vi "cam1analyse.vi"() -> (0 "W3 chiffre":string, 1 "W2 chiffre":string, 2 "R6 chiffre":string, 3 "W1 chiffre":string, 5 "W4 chiffre":string, 6 "B1 chiffre":string, 7 "B2 chiffre":string, 8 "R3 chiffre":string, 9 "R8 chiffre":string, 10 "B3 chiffre":string, 11 "B4 chiffre":string, 12 "B6 chiffre":string, 13 "B7 chiffre":string, 14 "B8 chiffre":string, 15 "B9 chiffre":string, 16 "R9 chiffre":string)   [LabVIEW 2019]
uses:
  <vilib>/vision/Classification.llb/IMAQ Classifier Read Options.ctl
  <vilib>/vision/NI_Vision_Development_Module.lvlib
panel:
  out "Coordinates":i32[](array[numeric])
  in  "R9":T1={"Global Rectangle"=[0, 0, 1279, 959], "Contours"=[{"ID"=enum."External", "Type"=3, "Coordinates"=[0, 0, 1279, 959]}]} {"Contours"."Type" items=["No Selection", "Point", "Line", "Rectangle", "Oval", "Polygon", "Freehand Region", "Annulus", "Unused2", "Unused3", "Broken Line", "Freehand Line", "Rotated Rectangle"]}
  out "R9 2":string[](array[string])
  in  "R8":T1={"Global Rectangle"=[0, 0, 1279, 959], "Contours"=[{"ID"=enum."External", "Type"=3, "Coordinates"=[0, 0, 1279, 959]}]} {"Contours"."Type" items=["No Selection", "Point", "Line", "Rectangle", "Oval", "Polygon", "Freehand Region", "Annulus", "Unused2", "Unused3", "Broken Line", "Freehand Line", "Rotated Rectangle"]}
  out "R8 2":string[](array[string])
  in  "R6":T1={"Global Rectangle"=[0, 0, 1279, 959], "Contours"=[{"ID"=enum."External", "Type"=3, "Coordinates"=[0, 0, 1279, 959]}]} {"Contours"."Type" items=["No Selection", "Point", "Line", "Rectangle", "Oval", "Polygon", "Freehand Region", "Annulus", "Unused2", "Unused3", "Broken Line", "Freehand Line", "Rotated Rectangle"]}
  out "R6 2":string[](array[string])
  in  "R3":T1={"Global Rectangle"=[0, 0, 1279, 959], "Contours"=[{"ID"=enum."External", "Type"=3, "Coordinates"=[0, 0, 1279, 959]}]} {"Contours"."Type" items=["No Selection", "Point", "Line", "Rectangle", "Oval", "Polygon", "Freehand Region", "Annulus", "Unused2", "Unused3", "Broken Line", "Freehand Line", "Rotated Rectangle"]}
  out "R3 2":string[](array[string])
  in  "B9":T1={"Global Rectangle"=[0, 0, 1279, 959], "Contours"=[{"ID"=enum."External", "Type"=3, "Coordinates"=[0, 0, 1279, 959]}]} {"Contours"."Type" items=["No Selection", "Point", "Line", "Rectangle", "Oval", "Polygon", "Freehand Region", "Annulus", "Unused2", "Unused3", "Broken Line", "Freehand Line", "Rotated Rectangle"]}
  out "B9 2":string[](array[string])
  in  "B8":T1={"Global Rectangle"=[0, 0, 1279, 959], "Contours"=[{"ID"=enum."External", "Type"=3, "Coordinates"=[0, 0, 1279, 959]}]} {"Contours"."Type" items=["No Selection", "Point", "Line", "Rectangle", "Oval", "Polygon", "Freehand Region", "Annulus", "Unused2", "Unused3", "Broken Line", "Freehand Line", "Rotated Rectangle"]}
  out "B8 2":string[](array[string])
  in  "B7":T1={"Global Rectangle"=[0, 0, 1279, 959], "Contours"=[{"ID"=enum."External", "Type"=3, "Coordinates"=[0, 0, 1279, 959]}]} {"Contours"."Type" items=["No Selection", "Point", "Line", "Rectangle", "Oval", "Polygon", "Freehand Region", "Annulus", "Unused2", "Unused3", "Broken Line", "Freehand Line", "Rotated Rectangle"]}
  out "B7 2":string[](array[string])
  in  "B6":T1={"Global Rectangle"=[0, 0, 1279, 959], "Contours"=[{"ID"=enum."External", "Type"=3, "Coordinates"=[0, 0, 1279, 959]}]} {"Contours"."Type" items=["No Selection", "Point", "Line", "Rectangle", "Oval", "Polygon", "Freehand Region", "Annulus", "Unused2", "Unused3", "Broken Line", "Freehand Line", "Rotated Rectangle"]}
  out "B6 2":string[](array[string])
  in  "B4":T1={"Global Rectangle"=[0, 0, 1279, 959], "Contours"=[{"ID"=enum."External", "Type"=3, "Coordinates"=[0, 0, 1279, 959]}]} {"Contours"."Type" items=["No Selection", "Point", "Line", "Rectangle", "Oval", "Polygon", "Freehand Region", "Annulus", "Unused2", "Unused3", "Broken Line", "Freehand Line", "Rotated Rectangle"]}
  out "B4 2":string[](array[string])
  in  "B3":T1={"Global Rectangle"=[0, 0, 1279, 959], "Contours"=[{"ID"=enum."External", "Type"=3, "Coordinates"=[0, 0, 1279, 959]}]} {"Contours"."Type" items=["No Selection", "Point", "Line", "Rectangle", "Oval", "Polygon", "Freehand Region", "Annulus", "Unused2", "Unused3", "Broken Line", "Freehand Line", "Rotated Rectangle"]}
  out "B3 2":string[](array[string])
  in  "B2":T1={"Global Rectangle"=[0, 0, 1279, 959], "Contours"=[{"ID"=enum."External", "Type"=3, "Coordinates"=[0, 0, 1279, 959]}]} {"Contours"."Type" items=["No Selection", "Point", "Line", "Rectangle", "Oval", "Polygon", "Freehand Region", "Annulus", "Unused2", "Unused3", "Broken Line", "Freehand Line", "Rotated Rectangle"]}
  out "B2 2":string[](array[string])
  in  "B1":T1={"Global Rectangle"=[0, 0, 1279, 959], "Contours"=[{"ID"=enum."External", "Type"=3, "Coordinates"=[0, 0, 1279, 959]}]} {"Contours"."Type" items=["No Selection", "Point", "Line", "Rectangle", "Oval", "Polygon", "Freehand Region", "Annulus", "Unused2", "Unused3", "Broken Line", "Freehand Line", "Rotated Rectangle"]}
  out "B1 2":string[](array[string])
  in  "W4":T1={"Global Rectangle"=[0, 0, 1279, 959], "Contours"=[{"ID"=enum."External", "Type"=3, "Coordinates"=[0, 0, 1279, 959]}]} {"Contours"."Type" items=["No Selection", "Point", "Line", "Rectangle", "Oval", "Polygon", "Freehand Region", "Annulus", "Unused2", "Unused3", "Broken Line", "Freehand Line", "Rotated Rectangle"]}
  out "W4 2":string[](array[string])
  in  "W1":T1={"Global Rectangle"=[0, 0, 1279, 959], "Contours"=[{"ID"=enum."External", "Type"=3, "Coordinates"=[0, 0, 1279, 959]}]} {"Contours"."Type" items=["No Selection", "Point", "Line", "Rectangle", "Oval", "Polygon", "Freehand Region", "Annulus", "Unused2", "Unused3", "Broken Line", "Freehand Line", "Rotated Rectangle"]}
  out "W1 2":string[](array[string])
  in  "W2 2":T1={"Global Rectangle"=[0, 0, 1279, 959], "Contours"=[{"ID"=enum."External", "Type"=3, "Coordinates"=[0, 0, 1279, 959]}]} {"Contours"."Type" items=["No Selection", "Point", "Line", "Rectangle", "Oval", "Polygon", "Freehand Region", "Annulus", "Unused2", "Unused3", "Broken Line", "Freehand Line", "Rotated Rectangle"]}
  out "W2 3":string[](array[string])
  in  "W3":T1={"Global Rectangle"=[640, 450, 686, 504], "Contours"=[{"ID"=enum."External", "Type"=3, "Coordinates"=[640, 450, 686, 504]}]} {"Contours"."Type" items=["No Selection", "Point", "Line", "Rectangle", "Oval", "Polygon", "Freehand Region", "Annulus", "Unused2", "Unused3", "Broken Line", "Freehand Line", "Rotated Rectangle"]}
  out "Image Out":T2(plugin-control)
  out "error out":errorcluster
  out "W3":string[](array[string])
  in  "error in":errorcluster
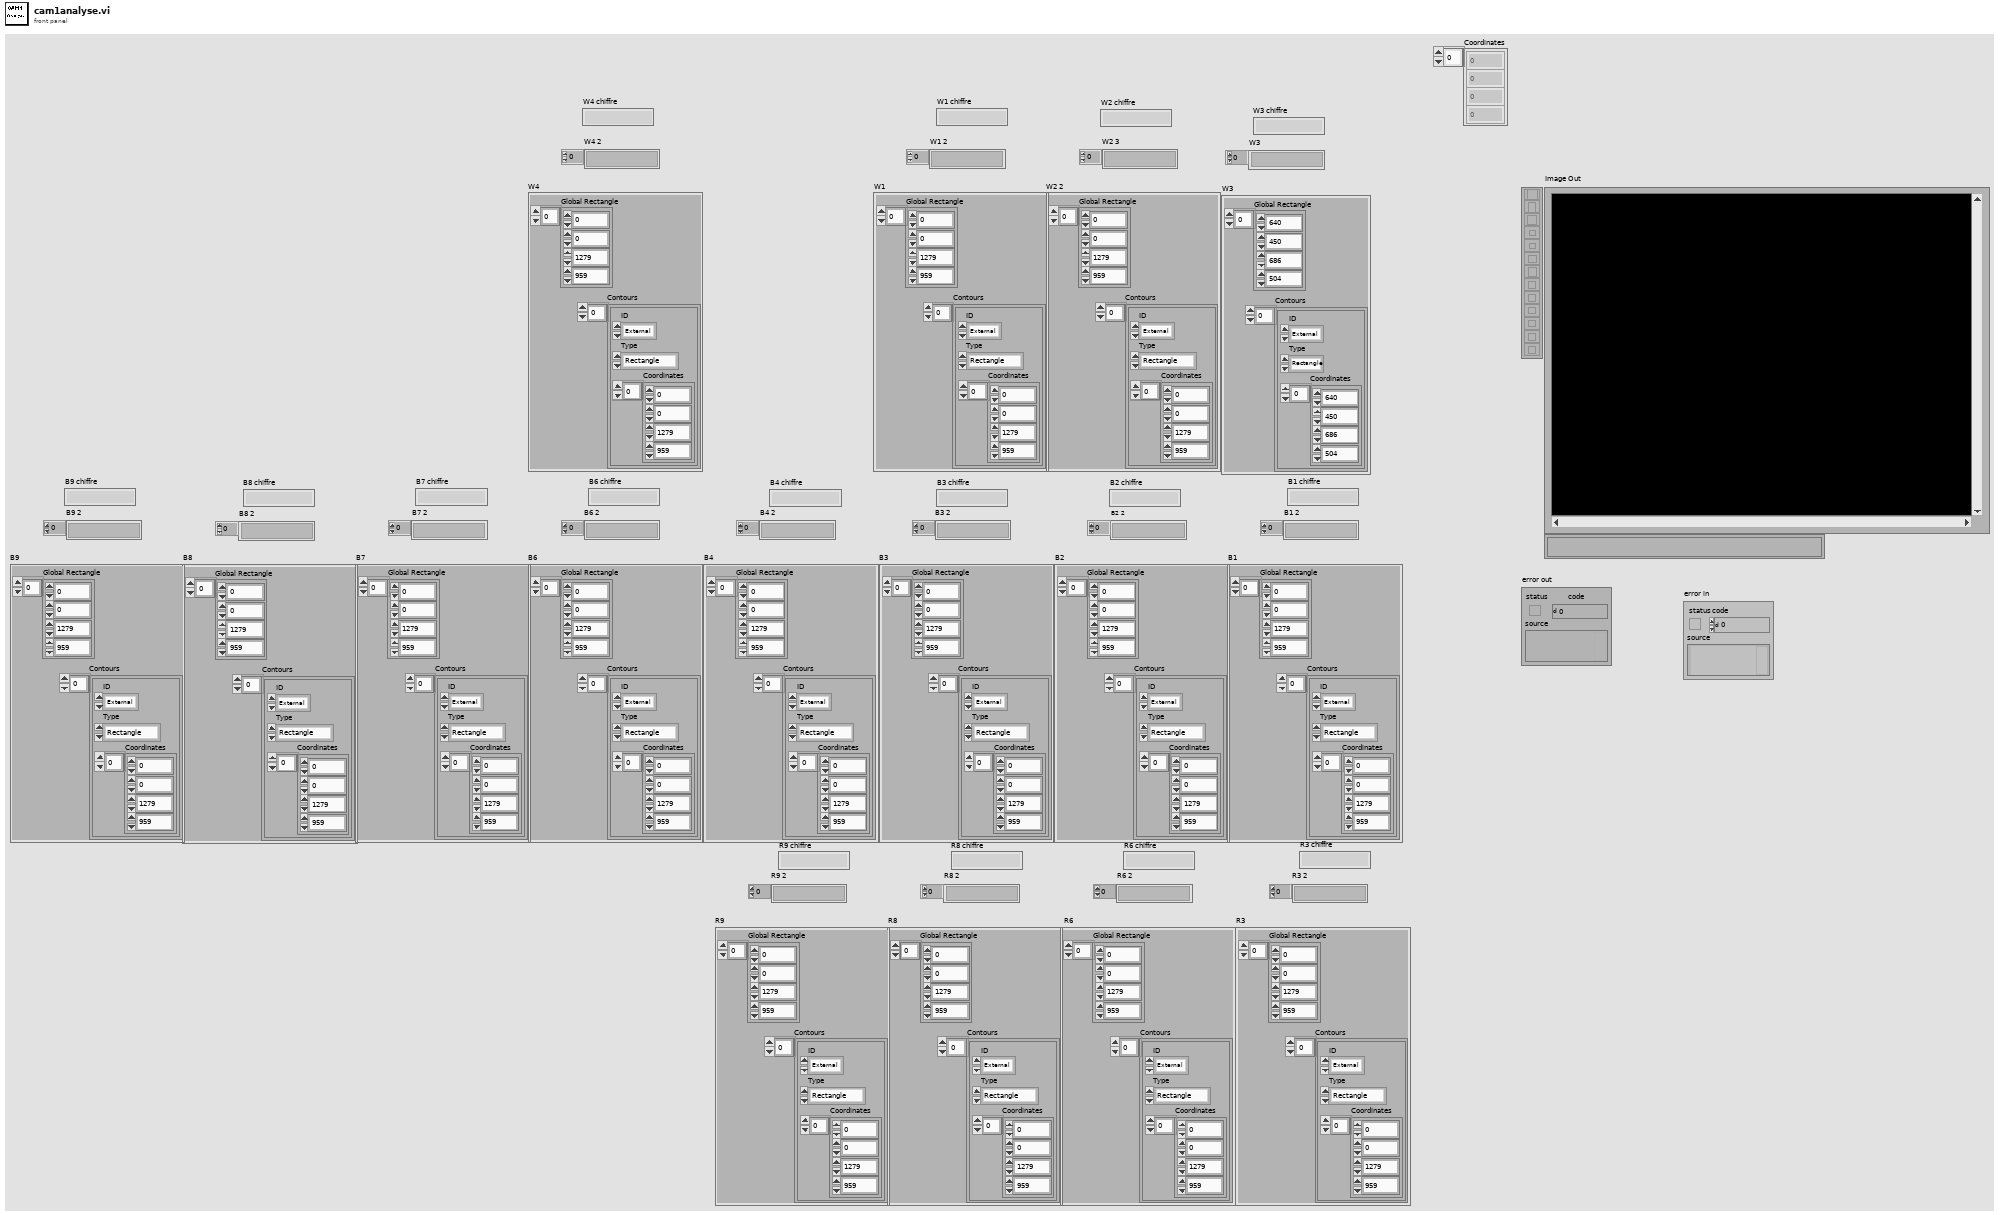
[diagram p1: front panel]
types:
  T1 = cluster{"Global Rectangle":i32[], "Contours":cluster{"ID":enum32{"External", "Internal"}, "Type":u32, "Coordinates":i32[]}[]}
  T2 = typedef "IMAQ Image.ctl" = refnum<image>
  T3 = typedef "IMAQ Classifier Read Options.ctl" = i32
  T4 = typedef "IMAQ Classifier Session.ctl" = refnum<k1>
  T5 = typedef "ROI Descriptor" = cluster{"Global Rectangle":i32[], "Contours":cluster{"ID":enum32{"External", "Internal"}, "Type":u32, "Coordinates":i32[]}[]}
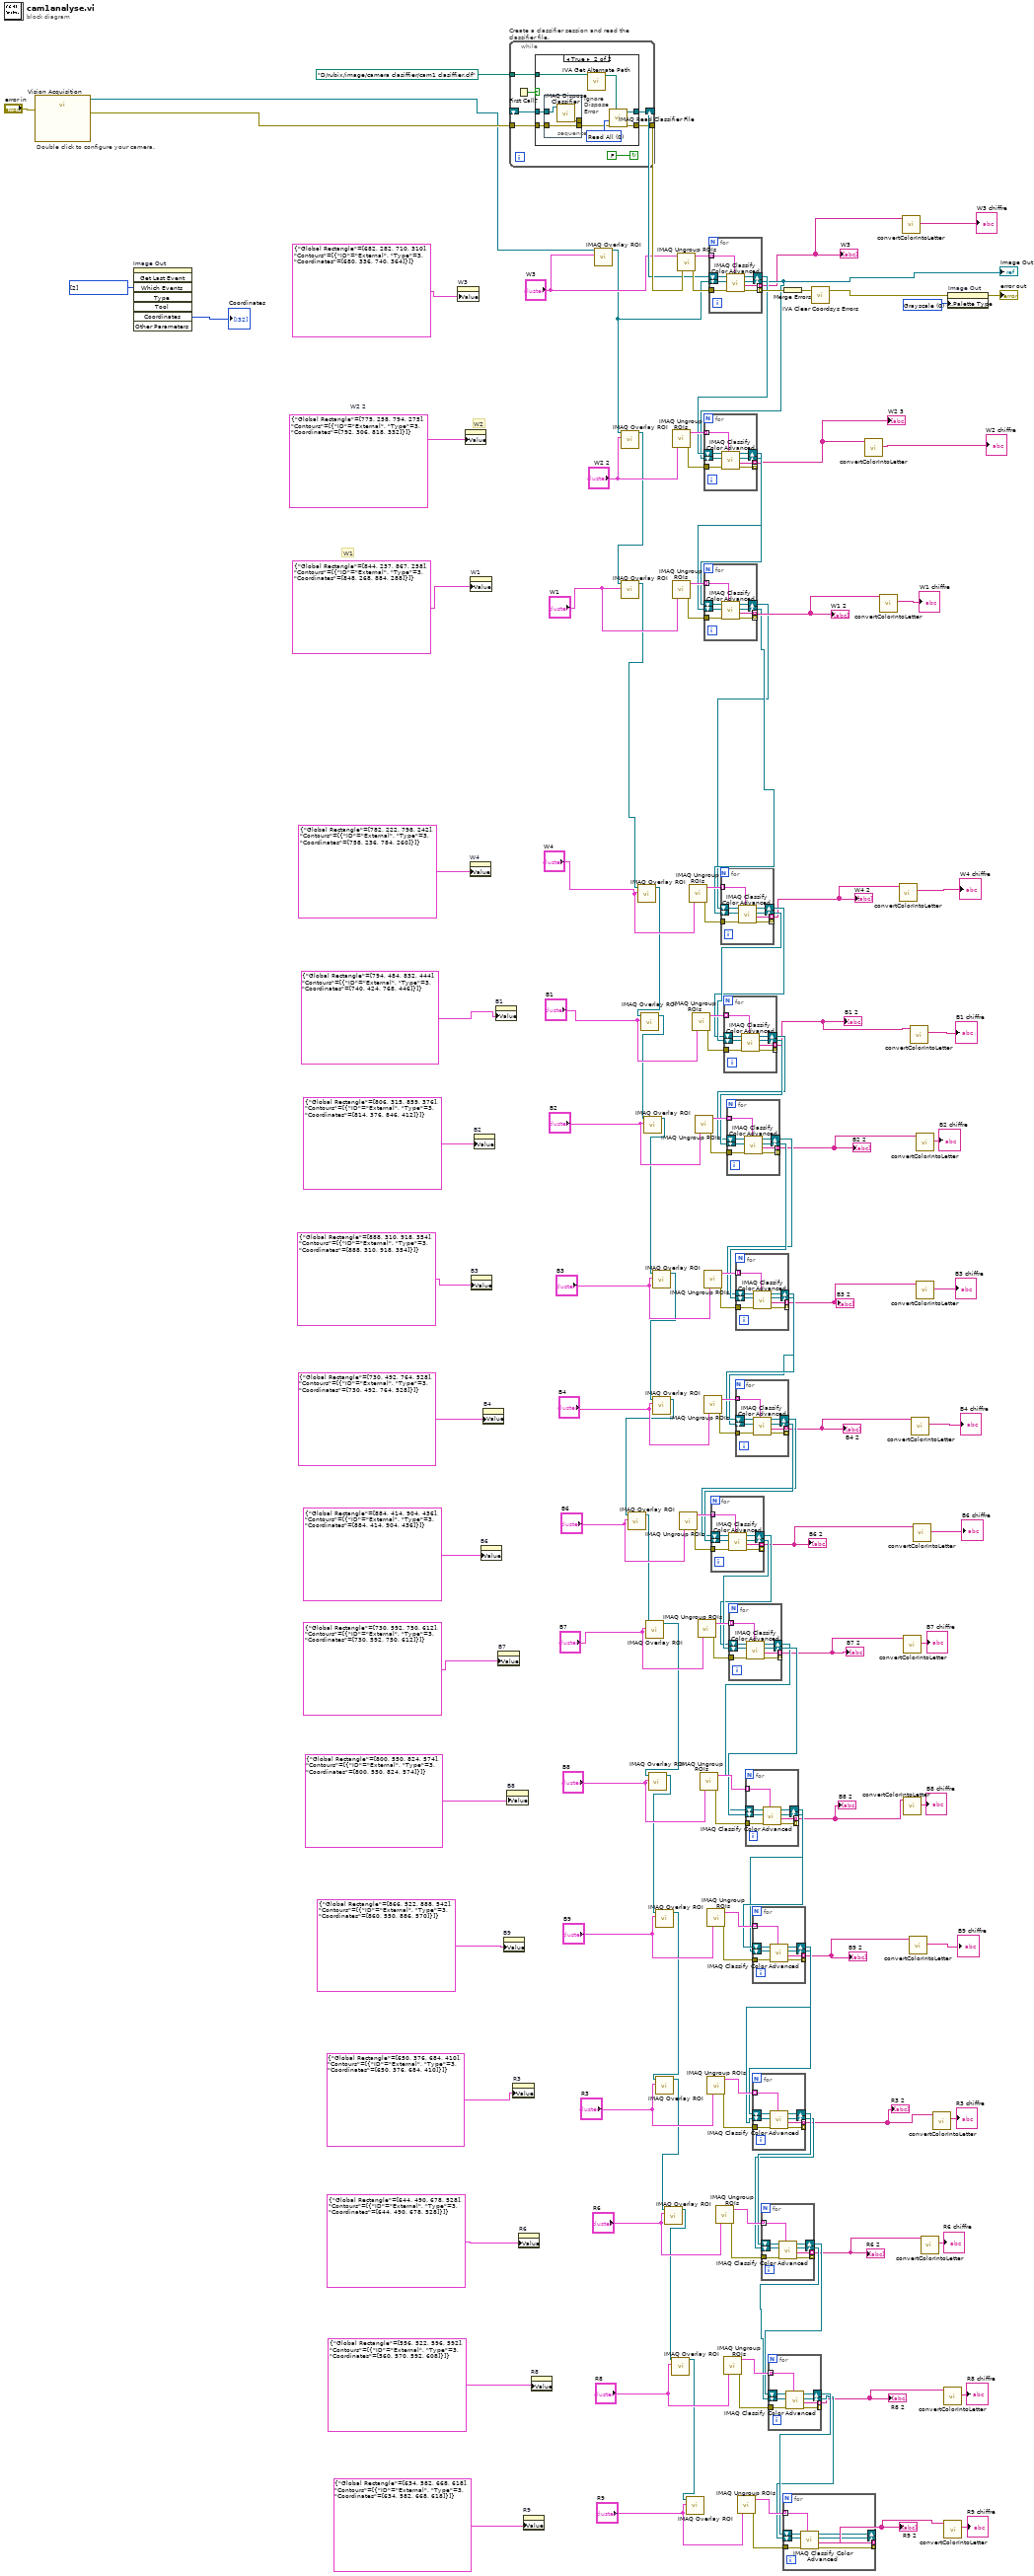
[diagram p0: block diagram]
diagram:
  w5 = i32[] [2] items=["No Event"=0, "Click Event"=1, "Draw Event"=2, "Size Event"=4, "Scroll Event"=5, "Double Click Event"=8] ("Which Events")
  w143 = u32 0 items=["Grayscale", "Binary", "Gradient", "Rainbow", "Temperature", "User Defined", "Binary 16 Bit", "Gradient 16 Bit", "Rainbow 16 Bit", "Temperature 16 Bit", "User Defined 16 Bit"] ("Palette Type")
  # "W2"
  # "W1"
  # "Double click to configure your camera."
  n1 = call "Vision Acquisition"("error in"="error in") -> ("Image Out"=w9:T2, "error out"=w153:errorcluster)  [unwired: 25 in]
  n2 = invoke on="Image Out" class="ImageControl" method="Get Last Event"("Which Events"=w5) -> ("Coordinates"=→"Coordinates":i32[])  [unwired: 7 in, 7 out]
  n3 = property on="W3" class="Clust (strict)"("Value"=T1 {"Global Rectangle"=[682, 282, 710, 310], "Contours"=[{"ID"=enum."External", "Type"=3, "Coordinates"=[680, 336, 740, 364]}]} ("ROI Descriptor (Color Classification 1)")) -> ()  [unwired: 2 in, 2 out]
  n4 = property on="W2 2" class="Clust (strict)"("Value"=T1 {"Global Rectangle"=[775, 258, 794, 275], "Contours"=[{"ID"=enum."External", "Type"=3, "Coordinates"=[792, 306, 818, 332]}]} ("ROI Descriptor (Color Classification 1)")) -> ()  [unwired: 2 in, 2 out]
  n5 = property on="W4" class="Clust (strict)"("Value"=T1 {"Global Rectangle"=[782, 222, 798, 242], "Contours"=[{"ID"=enum."External", "Type"=3, "Coordinates"=[758, 236, 784, 260]}]} ("ROI Descriptor (Color Classification 1)")) -> ()  [unwired: 2 in, 2 out]
  n6 = property on="W1" class="Clust (strict)"("Value"=T1 {"Global Rectangle"=[844, 237, 867, 258], "Contours"=[{"ID"=enum."External", "Type"=3, "Coordinates"=[848, 268, 884, 288]}]} ("ROI Descriptor (Color Classification 1)")) -> ()  [unwired: 2 in, 2 out]
  n7 = property on="B3" class="Clust (strict)"("Value"=T1 {"Global Rectangle"=[888, 310, 918, 354], "Contours"=[{"ID"=enum."External", "Type"=3, "Coordinates"=[888, 310, 918, 354]}]} ("ROI Descriptor (Color Classification 1)")) -> ()  [unwired: 2 in, 2 out]
  n8 = property on="B2" class="Clust (strict)"("Value"=T1 {"Global Rectangle"=[806, 315, 859, 376], "Contours"=[{"ID"=enum."External", "Type"=3, "Coordinates"=[814, 376, 846, 412]}]} ("ROI Descriptor (Color Classification 1)")) -> ()  [unwired: 2 in, 2 out]
  n9 = property on="B6" class="Clust (strict)"("Value"=T1 {"Global Rectangle"=[884, 414, 904, 436], "Contours"=[{"ID"=enum."External", "Type"=3, "Coordinates"=[884, 414, 904, 436]}]} ("ROI Descriptor (Color Classification 1)")) -> ()  [unwired: 2 in, 2 out]
  n10 = property on="B4" class="Clust (strict)"("Value"=T1 {"Global Rectangle"=[730, 492, 764, 528], "Contours"=[{"ID"=enum."External", "Type"=3, "Coordinates"=[730, 492, 764, 528]}]} ("ROI Descriptor (Color Classification 1)")) -> ()  [unwired: 2 in, 2 out]
  n11 = property on="B1" class="Clust (strict)"("Value"=T1 {"Global Rectangle"=[794, 484, 832, 444], "Contours"=[{"ID"=enum."External", "Type"=3, "Coordinates"=[740, 424, 768, 446]}]} ("ROI Descriptor (Color Classification 1)")) -> ()  [unwired: 2 in, 2 out]
  n12 = property on="B7" class="Clust (strict)"("Value"=T1 {"Global Rectangle"=[730, 592, 750, 612], "Contours"=[{"ID"=enum."External", "Type"=3, "Coordinates"=[730, 592, 750, 612]}]} ("ROI Descriptor (Color Classification 1)")) -> ()  [unwired: 2 in, 2 out]
  n13 = property on="B9" class="Clust (strict)"("Value"=T1 {"Global Rectangle"=[866, 522, 888, 542], "Contours"=[{"ID"=enum."External", "Type"=3, "Coordinates"=[860, 550, 886, 570]}]} ("ROI Descriptor (Color Classification 1)")) -> ()  [unwired: 2 in, 2 out]
  n14 = property on="B8" class="Clust (strict)"("Value"=T1 {"Global Rectangle"=[800, 550, 824, 574], "Contours"=[{"ID"=enum."External", "Type"=3, "Coordinates"=[800, 550, 824, 574]}]} ("ROI Descriptor (Color Classification 1)")) -> ()  [unwired: 2 in, 2 out]
  n15 = while "Create a classifier session and read the classifier file." {
    shift-right: [w161] -> w145
    shift-left: _ -> [w160]
    tunnel: w153 -> [w158]
    tunnel: [w157] -> w151
    tunnel: path "D:/rubix/image/camera clasiffier/cam1 clasiffier.clf" ("File Path") -> [w156]
    stop <- FALSE continue-if-true
    n16 = First Call?() -> (First Call?: T/F=w155:bool)
    n17 = case shown="True" w155 {
      tunnel: [w163 w170] -> w161
      tunnel: w160 -> [w163 w168]
      tunnel: w158 -> [w162 w167]
      tunnel: [w162 w169] -> w157
      tunnel: w156 -> [_ w165]
      frame False {
      }
      frame True {
        w171 = T3 0 items=["Read All", "Add Samples, Do Not Change Options", "Read Options, Do Not Add Samples"] ("Read Options")
        # "Ignore Dispose Error"
        n18 = stacked-sequence {
          tunnel: w168 -> [w174]
          tunnel: w167 -> [w173]
          tunnel: [w173] -> w166
          tunnel: [w172] -> _
          frame #0 {
            n19 = call "IMAQ Dispose Classifier"("Classifier Session"=w174) -> ("error out"=w172:errorcluster)  [unwired: 1 in, 9 out]
          }
        }
        n20 = call <vilib>:"IVA Get Alternate Path.vi"("Path In"=w165) -> ("Path Out"=w164:path)  [unwired: 10 out]
        n21 = call "IMAQ Read Classifier File"("File Path"=w164, "error in (no error)"=w166, "Read Options"=w171) -> ("error out"=w169:errorcluster, "Classifier Session"=w170:T4)  [unwired: 1 in, 6 out]
      }
    }
  }
  n22 = property on="R3" class="Clust (strict)"("Value"=T1 {"Global Rectangle"=[650, 376, 684, 410], "Contours"=[{"ID"=enum."External", "Type"=3, "Coordinates"=[650, 376, 684, 410]}]} ("ROI Descriptor (Color Classification 1)")) -> ()  [unwired: 2 in, 2 out]
  n23 = property on="R6" class="Clust (strict)"("Value"=T1 {"Global Rectangle"=[644, 490, 678, 528], "Contours"=[{"ID"=enum."External", "Type"=3, "Coordinates"=[644, 490, 678, 528]}]} ("ROI Descriptor (Color Classification 1)")) -> ()  [unwired: 2 in, 2 out]
  n24 = property on="R9" class="Clust (strict)"("Value"=T1 {"Global Rectangle"=[634, 582, 668, 618], "Contours"=[{"ID"=enum."External", "Type"=3, "Coordinates"=[634, 582, 668, 618]}]} ("ROI Descriptor (Color Classification 1)")) -> ()  [unwired: 2 in, 2 out]
  n25 = property on="R8" class="Clust (strict)"("Value"=T1 {"Global Rectangle"=[556, 522, 596, 592], "Contours"=[{"ID"=enum."External", "Type"=3, "Coordinates"=[560, 570, 592, 608]}]} ("ROI Descriptor (Color Classification 1)")) -> ()  [unwired: 2 in, 2 out]
  n26 = call "IMAQ Overlay ROI"("ROI Descriptor"="W3", "Image"=w9) -> ("Image Out"=w4:T2)  [unwired: 8 in, 1 out]
  n27 = call "IMAQ Overlay ROI"("ROI Descriptor"="W2 2", "Image"=w4) -> ("Image Out"=w136:T2)  [unwired: 8 in, 1 out]
  n28 = call "IMAQ Overlay ROI"("ROI Descriptor"="W1", "Image"=w136) -> ("Image Out"=w3:T2)  [unwired: 8 in, 1 out]
  n29 = call "IMAQ Overlay ROI"("ROI Descriptor"="W4", "Image"=w3) -> ("Image Out"=w123:T2)  [unwired: 8 in, 1 out]
  n30 = call "IMAQ Overlay ROI"("ROI Descriptor"="B1", "Image"=w123) -> ("Image Out"=w118:T2)  [unwired: 8 in, 1 out]
  n31 = call "IMAQ Overlay ROI"("ROI Descriptor"="B2", "Image"=w118) -> ("Image Out"=w111:T2)  [unwired: 8 in, 1 out]
  n32 = call "IMAQ Overlay ROI"("ROI Descriptor"="B3", "Image"=w111) -> ("Image Out"=w101:T2)  [unwired: 8 in, 1 out]
  n33 = call "IMAQ Overlay ROI"("ROI Descriptor"="B4", "Image"=w101) -> ("Image Out"=w97:T2)  [unwired: 8 in, 1 out]
  n34 = call "IMAQ Overlay ROI"("ROI Descriptor"="B6", "Image"=w97) -> ("Image Out"=w88:T2)  [unwired: 8 in, 1 out]
  n35 = call "IMAQ Overlay ROI"("ROI Descriptor"="B7", "Image"=w88) -> ("Image Out"=w83:T2)  [unwired: 8 in, 1 out]
  n36 = call "IMAQ Overlay ROI"("ROI Descriptor"="B8", "Image"=w83) -> ("Image Out"=w76:T2)  [unwired: 8 in, 1 out]
  n37 = call "IMAQ Overlay ROI"("ROI Descriptor"="B9", "Image"=w76) -> ("Image Out"=w69:T2)  [unwired: 8 in, 1 out]
  n38 = call "IMAQ Overlay ROI"("ROI Descriptor"="R3", "Image"=w69) -> ("Image Out"=w62:T2)  [unwired: 8 in, 1 out]
  n39 = call "IMAQ Overlay ROI"("ROI Descriptor"="R6", "Image"=w62) -> ("Image Out"=w55:T2)  [unwired: 8 in, 1 out]
  n40 = call "IMAQ Overlay ROI"("ROI Descriptor"="R8", "Image"=w55) -> ("Image Out"=w48:T2)  [unwired: 8 in, 1 out]
  n41 = call "IMAQ Ungroup ROIs"("ROI Descriptor"="W2 2") -> ("error out"=w142:errorcluster, "ROI Descriptors out"=w141:T5[])  [unwired: 1 in, 2 out]
  n42 = call "IMAQ Ungroup ROIs"("ROI Descriptor"="W1") -> ("error out"=w138:errorcluster, "ROI Descriptors out"=w137:T5[])  [unwired: 1 in, 2 out]
  n43 = call "IMAQ Ungroup ROIs"("error in (no error)"=w151, "ROI Descriptor"="W3") -> ("error out"=w150:errorcluster, "ROI Descriptors out"=w149:T5[])  [unwired: 2 out]
  n44 = call "IMAQ Ungroup ROIs"("ROI Descriptor"="B6") -> ("error out"=w100:errorcluster, "ROI Descriptors out"=w99:T5[])  [unwired: 1 in, 2 out]
  n45 = call "IMAQ Overlay ROI"("ROI Descriptor"="R9", "Image"=w48) -> ()  [unwired: 8 in, 2 out]
  n46 = call "IMAQ Ungroup ROIs"("ROI Descriptor"="W4") -> ("error out"=w131:errorcluster, "ROI Descriptors out"=w130:T5[])  [unwired: 1 in, 2 out]
  n47 = call "IMAQ Ungroup ROIs"("ROI Descriptor"="B1") -> ("error out"=w127:errorcluster, "ROI Descriptors out"=w126:T5[])  [unwired: 1 in, 2 out]
  n48 = call "IMAQ Ungroup ROIs"("ROI Descriptor"="B2") -> ("error out"=w121:errorcluster, "ROI Descriptors out"=w120:T5[])  [unwired: 1 in, 2 out]
  n49 = call "IMAQ Ungroup ROIs"("ROI Descriptor"="B7") -> ("error out"=w93:errorcluster, "ROI Descriptors out"=w92:T5[])  [unwired: 1 in, 2 out]
  n50 = call "IMAQ Ungroup ROIs"("ROI Descriptor"="B8") -> ("error out"=w86:errorcluster, "ROI Descriptors out"=w85:T5[])  [unwired: 1 in, 2 out]
  n51 = call "IMAQ Ungroup ROIs"("ROI Descriptor"="B4") -> ("error out"=w107:errorcluster, "ROI Descriptors out"=w106:T5[])  [unwired: 1 in, 2 out]
  n52 = call "IMAQ Ungroup ROIs"("ROI Descriptor"="B3") -> ("error out"=w114:errorcluster, "ROI Descriptors out"=w113:T5[])  [unwired: 1 in, 2 out]
  n53 = call "IMAQ Ungroup ROIs"("ROI Descriptor"="B9") -> ("error out"=w79:errorcluster, "ROI Descriptors out"=w78:T5[])  [unwired: 1 in, 2 out]
  n54 = call "IMAQ Ungroup ROIs"("ROI Descriptor"="R3") -> ("error out"=w72:errorcluster, "ROI Descriptors out"=w71:T5[])  [unwired: 1 in, 2 out]
  n55 = for {
    tunnel: [w182] -> w12 mode=indexing
    tunnel: [w181] -> w148 mode=indexing
    tunnel: w150 -> [w179]
    tunnel: w149 -> [w178] mode=indexing
    shift-right: [w176] -> w14
    shift-left: w4 -> [w177]
    shift-right: [w175] -> w15
    shift-left: w145 -> [w180]
    n56 = call "IMAQ Classify Color Advanced"("ROI Descriptor"=w178, "error in (no error)"=w179, "Image"=w177, "Classifier Session"=w180) -> ("error out"=w181:errorcluster, "Class"=w182:string, "Image (dup)"=w176:T2, "Classifier Session (dup)"=w175:T4)  [unwired: 4 out]
  }
  "W3" <- w12
  "Image Out" <- w14
  n57 = for {
    tunnel: [w190] -> w8 mode=indexing
    tunnel: [w189] -> _ mode=indexing
    tunnel: w142 -> [w187]
    tunnel: w141 -> [w186] mode=indexing
    shift-right: [w184] -> w134
    shift-left: w14 -> [w185]
    shift-right: [w183] -> w135
    shift-left: w15 -> [w188]
    n58 = call "IMAQ Classify Color Advanced"("ROI Descriptor"=w186, "error in (no error)"=w187, "Image"=w185, "Classifier Session"=w188) -> ("error out"=w189:errorcluster, "Class"=w190:string, "Image (dup)"=w184:T2, "Classifier Session (dup)"=w183:T4)  [unwired: 4 out]
  }
  "W2 3" <- w8
  n59 = for {
    tunnel: [w198] -> w43 mode=indexing
    tunnel: [w197] -> _ mode=indexing
    tunnel: w138 -> [w195]
    tunnel: w137 -> [w194] mode=indexing
    shift-right: [w192] -> w2
    shift-left: w134 -> [w193]
    shift-right: [w191] -> w1
    shift-left: w135 -> [w196]
    n60 = call "IMAQ Classify Color Advanced"("ROI Descriptor"=w194, "error in (no error)"=w195, "Image"=w193, "Classifier Session"=w196) -> ("error out"=w197:errorcluster, "Class"=w198:string, "Image (dup)"=w192:T2, "Classifier Session (dup)"=w191:T4)  [unwired: 4 out]
  }
  "W1 2" <- w43
  n61 = call "IMAQ Ungroup ROIs"("ROI Descriptor"="R6") -> ("error out"=w65:errorcluster, "ROI Descriptors out"=w64:T5[])  [unwired: 1 in, 2 out]
  n62 = for {
    tunnel: [w206] -> w42 mode=indexing
    tunnel: [w205] -> _ mode=indexing
    tunnel: w131 -> [w203]
    tunnel: w130 -> [w202] mode=indexing
    shift-right: [w200] -> w125
    shift-left: w2 -> [w201]
    shift-right: [w199] -> w124
    shift-left: w1 -> [w204]
    n63 = call "IMAQ Classify Color Advanced"("ROI Descriptor"=w202, "error in (no error)"=w203, "Image"=w201, "Classifier Session"=w204) -> ("error out"=w205:errorcluster, "Class"=w206:string, "Image (dup)"=w200:T2, "Classifier Session (dup)"=w199:T4)  [unwired: 4 out]
  }
  "W4 2" <- w42
  n64 = call "IMAQ Ungroup ROIs"("ROI Descriptor"="R8") -> ("error out"=w58:errorcluster, "ROI Descriptors out"=w57:T5[])  [unwired: 1 in, 2 out]
  n65 = for {
    tunnel: [w214] -> w41 mode=indexing
    tunnel: [w213] -> _ mode=indexing
    tunnel: w127 -> [w211]
    tunnel: w126 -> [w210] mode=indexing
    shift-right: [w208] -> w117
    shift-left: w125 -> [w209]
    shift-right: [w207] -> w116
    shift-left: w124 -> [w212]
    n66 = call "IMAQ Classify Color Advanced"("ROI Descriptor"=w210, "error in (no error)"=w211, "Image"=w209, "Classifier Session"=w212) -> ("error out"=w213:errorcluster, "Class"=w214:string, "Image (dup)"=w208:T2, "Classifier Session (dup)"=w207:T4)  [unwired: 4 out]
  }
  "B1 2" <- w41
  n67 = for {
    tunnel: [w222] -> w40 mode=indexing
    tunnel: [w221] -> _ mode=indexing
    tunnel: w121 -> [w219]
    tunnel: w120 -> [w218] mode=indexing
    shift-right: [w216] -> w110
    shift-left: w117 -> [w217]
    shift-right: [w215] -> w109
    shift-left: w116 -> [w220]
    n68 = call "IMAQ Classify Color Advanced"("ROI Descriptor"=w218, "error in (no error)"=w219, "Image"=w217, "Classifier Session"=w220) -> ("error out"=w221:errorcluster, "Class"=w222:string, "Image (dup)"=w216:T2, "Classifier Session (dup)"=w215:T4)  [unwired: 4 out]
  }
  "B2 2" <- w40
  n69 = for {
    tunnel: [w230] -> w39 mode=indexing
    tunnel: [w229] -> _ mode=indexing
    tunnel: w114 -> [w227]
    tunnel: w113 -> [w226] mode=indexing
    shift-right: [w224] -> w104
    shift-left: w110 -> [w225]
    shift-right: [w223] -> w105
    shift-left: w109 -> [w228]
    n70 = call "IMAQ Classify Color Advanced"("ROI Descriptor"=w226, "error in (no error)"=w227, "Image"=w225, "Classifier Session"=w228) -> ("error out"=w229:errorcluster, "Class"=w230:string, "Image (dup)"=w224:T2, "Classifier Session (dup)"=w223:T4)  [unwired: 4 out]
  }
  "B3 2" <- w39
  n71 = for {
    tunnel: [w238] -> w38 mode=indexing
    tunnel: [w237] -> _ mode=indexing
    tunnel: w107 -> [w235]
    tunnel: w106 -> [w234] mode=indexing
    shift-right: [w232] -> w96
    shift-left: w104 -> [w233]
    shift-right: [w231] -> w95
    shift-left: w105 -> [w236]
    n72 = call "IMAQ Classify Color Advanced"("ROI Descriptor"=w234, "error in (no error)"=w235, "Image"=w233, "Classifier Session"=w236) -> ("error out"=w237:errorcluster, "Class"=w238:string, "Image (dup)"=w232:T2, "Classifier Session (dup)"=w231:T4)  [unwired: 4 out]
  }
  "B4 2" <- w38
  n73 = for {
    tunnel: [w246] -> w37 mode=indexing
    tunnel: [w245] -> _ mode=indexing
    tunnel: w100 -> [w243]
    tunnel: w99 -> [w242] mode=indexing
    shift-right: [w240] -> w91
    shift-left: w96 -> [w241]
    shift-right: [w239] -> w90
    shift-left: w95 -> [w244]
    n74 = call "IMAQ Classify Color Advanced"("ROI Descriptor"=w242, "error in (no error)"=w243, "Image"=w241, "Classifier Session"=w244) -> ("error out"=w245:errorcluster, "Class"=w246:string, "Image (dup)"=w240:T2, "Classifier Session (dup)"=w239:T4)  [unwired: 4 out]
  }
  "B6 2" <- w37
  n75 = for {
    tunnel: [w254] -> w36 mode=indexing
    tunnel: [w253] -> _ mode=indexing
    tunnel: w93 -> [w251]
    tunnel: w92 -> [w250] mode=indexing
    shift-right: [w248] -> w82
    shift-left: w91 -> [w249]
    shift-right: [w247] -> w81
    shift-left: w90 -> [w252]
    n76 = call "IMAQ Classify Color Advanced"("ROI Descriptor"=w250, "error in (no error)"=w251, "Image"=w249, "Classifier Session"=w252) -> ("error out"=w253:errorcluster, "Class"=w254:string, "Image (dup)"=w248:T2, "Classifier Session (dup)"=w247:T4)  [unwired: 4 out]
  }
  "B7 2" <- w36
  n77 = call "IMAQ Ungroup ROIs"("ROI Descriptor"="R9") -> ("error out"=w51:errorcluster, "ROI Descriptors out"=w50:T5[])  [unwired: 1 in, 2 out]
  n78 = for {
    tunnel: [w262] -> w35 mode=indexing
    tunnel: [w261] -> _ mode=indexing
    tunnel: w86 -> [w259]
    tunnel: w85 -> [w258] mode=indexing
    shift-right: [w256] -> w74
    shift-left: w82 -> [w257]
    shift-right: [w255] -> w75
    shift-left: w81 -> [w260]
    n79 = call "IMAQ Classify Color Advanced"("ROI Descriptor"=w258, "error in (no error)"=w259, "Image"=w257, "Classifier Session"=w260) -> ("error out"=w261:errorcluster, "Class"=w262:string, "Image (dup)"=w256:T2, "Classifier Session (dup)"=w255:T4)  [unwired: 4 out]
  }
  "B8 2" <- w35
  n80 = for {
    tunnel: [w270] -> w34 mode=indexing
    tunnel: [w269] -> _ mode=indexing
    tunnel: w79 -> [w267]
    tunnel: w78 -> [w266] mode=indexing
    shift-right: [w264] -> w67
    shift-left: w74 -> [w265]
    shift-right: [w263] -> w68
    shift-left: w75 -> [w268]
    n81 = call "IMAQ Classify Color Advanced"("ROI Descriptor"=w266, "error in (no error)"=w267, "Image"=w265, "Classifier Session"=w268) -> ("error out"=w269:errorcluster, "Class"=w270:string, "Image (dup)"=w264:T2, "Classifier Session (dup)"=w263:T4)  [unwired: 4 out]
  }
  "B9 2" <- w34
  n82 = for {
    tunnel: [w278] -> w33 mode=indexing
    tunnel: [w277] -> _ mode=indexing
    tunnel: w72 -> [w275]
    tunnel: w71 -> [w274] mode=indexing
    shift-right: [w272] -> w60
    shift-left: w67 -> [w273]
    shift-right: [w271] -> w61
    shift-left: w68 -> [w276]
    n83 = call "IMAQ Classify Color Advanced"("ROI Descriptor"=w274, "error in (no error)"=w275, "Image"=w273, "Classifier Session"=w276) -> ("error out"=w277:errorcluster, "Class"=w278:string, "Image (dup)"=w272:T2, "Classifier Session (dup)"=w271:T4)  [unwired: 4 out]
  }
  "R3 2" <- w33
  n84 = for {
    tunnel: [w286] -> w32 mode=indexing
    tunnel: [w285] -> _ mode=indexing
    tunnel: w65 -> [w283]
    tunnel: w64 -> [w282] mode=indexing
    shift-right: [w280] -> w54
    shift-left: w60 -> [w281]
    shift-right: [w279] -> w53
    shift-left: w61 -> [w284]
    n85 = call "IMAQ Classify Color Advanced"("ROI Descriptor"=w282, "error in (no error)"=w283, "Image"=w281, "Classifier Session"=w284) -> ("error out"=w285:errorcluster, "Class"=w286:string, "Image (dup)"=w280:T2, "Classifier Session (dup)"=w279:T4)  [unwired: 4 out]
  }
  "R6 2" <- w32
  n86 = for {
    tunnel: [w294] -> w31 mode=indexing
    tunnel: [w293] -> _ mode=indexing
    tunnel: w58 -> [w291]
    tunnel: w57 -> [w290] mode=indexing
    shift-right: [w288] -> w46
    shift-left: w54 -> [w289]
    shift-right: [w287] -> w47
    shift-left: w53 -> [w292]
    n87 = call "IMAQ Classify Color Advanced"("ROI Descriptor"=w290, "error in (no error)"=w291, "Image"=w289, "Classifier Session"=w292) -> ("error out"=w293:errorcluster, "Class"=w294:string, "Image (dup)"=w288:T2, "Classifier Session (dup)"=w287:T4)  [unwired: 4 out]
  }
  "R8 2" <- w31
  n88 = for {
    tunnel: [w302] -> w30 mode=indexing
    tunnel: [w301] -> _ mode=indexing
    tunnel: w51 -> [w299]
    tunnel: w50 -> [w298] mode=indexing
    shift-right: [w296] -> _
    shift-left: w46 -> [w297]
    shift-right: [w295] -> _
    shift-left: w47 -> [w300]
    n89 = call "IMAQ Classify Color Advanced"("ROI Descriptor"=w298, "error in (no error)"=w299, "Image"=w297, "Classifier Session"=w300) -> ("error out"=w301:errorcluster, "Class"=w302:string, "Image (dup)"=w296:T2, "Classifier Session (dup)"=w295:T4)  [unwired: 4 out]
  }
  "R9 2" <- w30
  n90 = Merge Errors(w148) -> (w147:errorcluster)
  n91 = call <vilib>:"IVA Clear Coordsys Errors.vi"("error in (no error)"=w147) -> ("error out"=w146:errorcluster)  [unwired: 10 in]
  n92 = call "convertColorIntoLetter.vi"("Array"=w8) -> ("String"=→"W2 chiffre":string)  [unwired: 10 in]
  n93 = call "convertColorIntoLetter.vi"("Array"=w43) -> ("String"=→"W1 chiffre":string)  [unwired: 10 in]
  n94 = call "convertColorIntoLetter.vi"("Array"=w42) -> ("String"=→"W4 chiffre":string)  [unwired: 10 in]
  n95 = call "convertColorIntoLetter.vi"("Array"=w12) -> ("String"=→"W3 chiffre":string)  [unwired: 10 in]
  n96 = call "convertColorIntoLetter.vi"("Array"=w35) -> ("String"=→"B8 chiffre":string)  [unwired: 10 in]
  n97 = call "convertColorIntoLetter.vi"("Array"=w36) -> ("String"=→"B7 chiffre":string)  [unwired: 10 in]
  n98 = call "convertColorIntoLetter.vi"("Array"=w34) -> ("String"=→"B9 chiffre":string)  [unwired: 10 in]
  n99 = call "convertColorIntoLetter.vi"("Array"=w41) -> ("String"=→"B1 chiffre":string)  [unwired: 10 in]
  n100 = call "convertColorIntoLetter.vi"("Array"=w38) -> ("String"=→"B4 chiffre":string)  [unwired: 10 in]
  n101 = call "convertColorIntoLetter.vi"("Array"=w37) -> ("String"=→"B6 chiffre":string)  [unwired: 10 in]
  n102 = call "convertColorIntoLetter.vi"("Array"=w40) -> ("String"=→"B2 chiffre":string)  [unwired: 10 in]
  n103 = call "convertColorIntoLetter.vi"("Array"=w39) -> ("String"=→"B3 chiffre":string)  [unwired: 10 in]
  n104 = call "convertColorIntoLetter.vi"("Array"=w32) -> ("String"=→"R6 chiffre":string)  [unwired: 10 in]
  n105 = call "convertColorIntoLetter.vi"("Array"=w33) -> ("String"=→"R3 chiffre":string)  [unwired: 10 in]
  n106 = call "convertColorIntoLetter.vi"("Array"=w31) -> ("String"=→"R8 chiffre":string)  [unwired: 10 in]
  n107 = call "convertColorIntoLetter.vi"("Array"=w30) -> ("String"=→"R9 chiffre":string)  [unwired: 10 in]
  n108 = property on="Image Out" class="ImageControl"(error in=w146, "Palette:Palette Type"=w143) -> (error out=→"error out":errorcluster)  [unwired: 1 in, 1 out]
